vi "GraspMapTHIN_sensorFrame.vi"() -> (0 "Grasp Map":T1)   [LabVIEW 2021]
uses:
  <vilib>/Analysis/Matrix/Datatypes/RealMatrix.ctl
  <vilib>/Analysis/baseanly.llb/Real A x B.vi
  <vilib>/Analysis/Matrix/NI_Matrix.lvlib
  <vilib>/Analysis/NI_AALBase.lvlib
panel:
  in  "half handle width (m)":dbl=0.0216
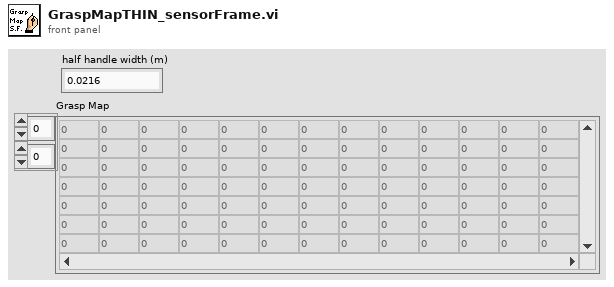
[diagram p1: front panel]
types:
  T1 = typedef "NI_Matrix.lvlib/RealMatrix.ctl" = dbl[][]
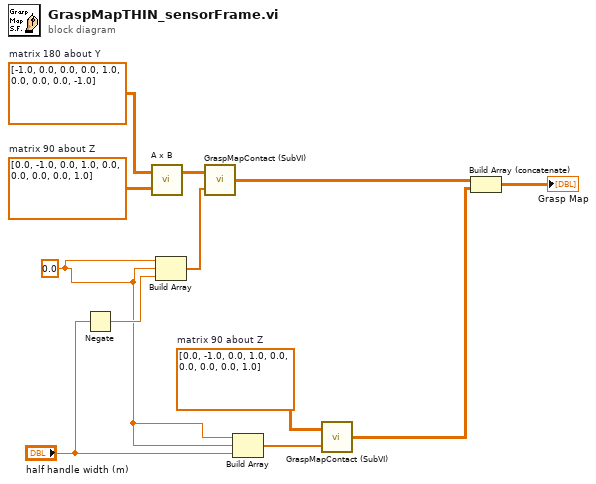
[diagram p0: block diagram]
diagram:
  w1 = 0.0 ("element")
  w7 = T1 [[0.0, -1.0, 0.0], [1.0, 0.0, 0.0], [0.0, 0.0, 1.0]]  # matrix 90 about Z
  w8 = T1 [[0.0, -1.0, 0.0], [1.0, 0.0, 0.0], [0.0, 0.0, 1.0]]  # matrix 90 about Z
  w6 = T1 [[-1.0, 0.0, 0.0], [0.0, 1.0, 0.0], [0.0, 0.0, -1.0]]  # matrix 180 about Y
  n1 = Negate(x="half handle width (m)") -> (-x=w5:dbl)
  n2 = call-poly <vilib>:"A x B.vi"("B"=w8, "A"=w6) -> ("A x B"=w9:T1)  [unwired: 1 out]
  n3 = Build Array(w1, w1, w5) -> (w4:dbl[])
  n4 = call "GraspMapContact (SubVI).vi"("position Vector"=w4, "r matrix"=w9) -> ("contact grasp map matrix"=w12:T1)
  n5 = Build Array(w1, w1, "half handle width (m)") -> (w2:dbl[])
  n6 = call "GraspMapContact (SubVI).vi"("position Vector"=w2, "r matrix"=w7) -> ("contact grasp map matrix"=w11:T1)
  n7 = Build Array (concatenate) ("Build Matrix")(w12, w11) -> (→"Grasp Map":T1)
